vi "Stop Core.vi"(10 "final error code":i32, 11 "UDP_receiver in":refnum<class "UDP_receiver.lvclass">) -> (3 "UDP_receiver out":refnum<class "UDP_receiver.lvclass">)   [LabVIEW 2025, in "UDP_receiver.lvlib" / "UDP_receiver.lvclass"]
doc: "(<B>Filename</B>: Actor Framework.lvlib:Actor.lvclass:Stop Core.vi)\n\nDefines what the actor does before it stops. Use the <B>final error code</B> input to determine whether the actor shut down in response to an error.\n\nBy default, this method passes the Stop message along to all auto-stop nested actors. A descendant class may override this method to define additional behavior, such as shutting down any processes the actor initiated in its override of the Actor Core method."
uses:
  UDP_receiver.lvclass
  C:/Program Files/National Instruments/LabVIEW 2025/vi.lib/ActorFramework/Actor/Actor.lvclass
  <vilib>/ActorFramework/Actor/Actor.lvclass/Actor.ctl
  UDP_receiver.lvclass/UDP_receiver.ctl
  <vilib>/ActorFramework/Message Enqueuer/Message Enqueuer.lvclass/Message Enqueuer.ctl
  <vilib>/ActorFramework/Message Enqueuer/Enqueue.vi
  root_actor/root_actor Messages/stop_app1 Msg/stop_app1 Msg.lvclass
  C:/Program Files/National Instruments/LabVIEW 2025/vi.lib/ActorFramework/Message/Message.lvclass
  <vilib>/ActorFramework/Message Priority Queue/Priority Enqueue.vi
  <vilib>/ActorFramework/Actor/Actor.lvclass
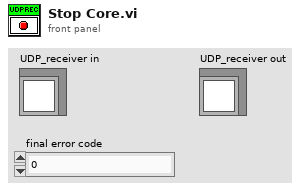
[diagram p1: front panel]
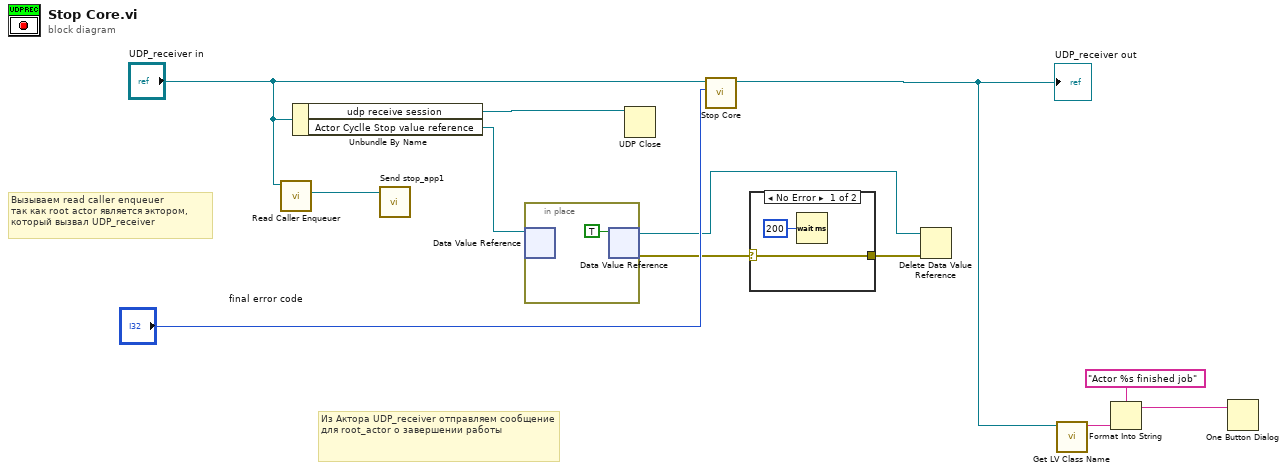
[diagram p0: block diagram]
diagram:
  # "Вызываем read caller enqueuer\nтак как root actor является эктором, \nкоторый вызвал UDP_receiver"
  # "Из Актора UDP_receiver отправляем сообщение \nдля root_actor о завершении работы"
  n1 = call <vilib>:"Read Caller Enqueuer.vi"("Actor"="UDP_receiver in") -> ("Caller Enqueuer"=w5:refnum<class "Message Enqueuer.lvclass">)  [unwired: 10 in]
  n2 = Unbundle By Name("UDP_receiver in") -> ("udp receive session"=w11:refnum<k16>, "Actor Cyclle Stop value reference"=w10:refnum<data-value>)
  n3 = call "Send stop_app1.vi"("Message Enqueuer"=w5) -> ()  [unwired: 9 in, 2 out]
  n4 = in-place {
    n5 = in-place-dvr #1(w10) -> ()  [unwired: 2 out]
    n6 = in-place-dvr #1(TRUE ("data value")) -> (w7:refnum<data-value>, w9:errorcluster)
  }
  n7 = UDP Close(connection ID=w11) -> ()  [unwired: 1 in, 2 out]
  n8 = call-parent "Stop Core.vi"("final error code"="final error code", "Actor in"="UDP_receiver in") -> ("Actor out"=w1:refnum<class "UDP_receiver.lvclass">)  [unwired: 9 in]
  "UDP_receiver out" <- w1
  n9 = case shown="No Error" w9 {
    selector: w9 -> [w14 w16]
    tunnel: [w14 w16] -> w8
    frame No Error {
      n10 = Wait (ms)(milliseconds to wait=u32 200) -> ()  [unwired: 1 out]
    }
    frame Error {
    }
  }
  n11 = Delete Data Value Reference(data value reference=w7, error in=w8) -> ()  [unwired: 2 out]
  n12 = call <vilib>:"Get LV Class Name.vi"("object"=w1) -> ("class name"=w4:string)  [unwired: 9 in, 1 out]
  n13 = Format Into String(format string="Actor %s finished job", w4) -> (resulting string=w2:string)  [unwired: 2 in, 1 out]
  n14 = One Button Dialog(message=w2) -> ()  [unwired: 1 in, 1 out]
